vi "Formal Check Squares by Int.vi"(10 "Sudoku Formal In":T1, 11 "Sudoku Int":u8[][](array[numeric])) -> (2 "Sudoku Formal Out":T1, 3 "Is Modify":bool)   [LabVIEW 2015, in "Sudoku Library.lvlib"]
doc: "Created IvanLis by LabVIEW Portal\nProfile: http://labviewportal.org/memberlist.php?mode=viewprofile&u=987\neMail: IvanLisanov@gMail.com\nTelegram: https://t.me/IvanLis"
uses:
  Sudoku Library.lvlib
  TypeDef/Sudoku Formal.ctl
  TypeDef/Cell Formal.ctl
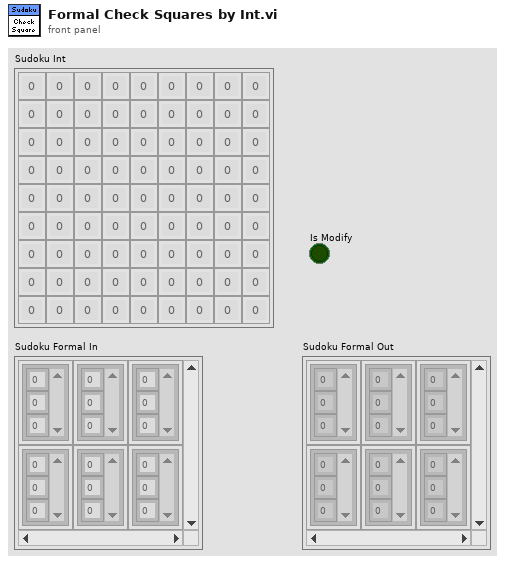
[diagram p1: front panel]
types:
  T1 = typedef "Sudoku Library.lvlib/Sudoku Formal.ctl" = T2[][]
  T2 = typedef "Sudoku Library.lvlib/Cell Formal.ctl" = cluster{"Variant":u8[]}
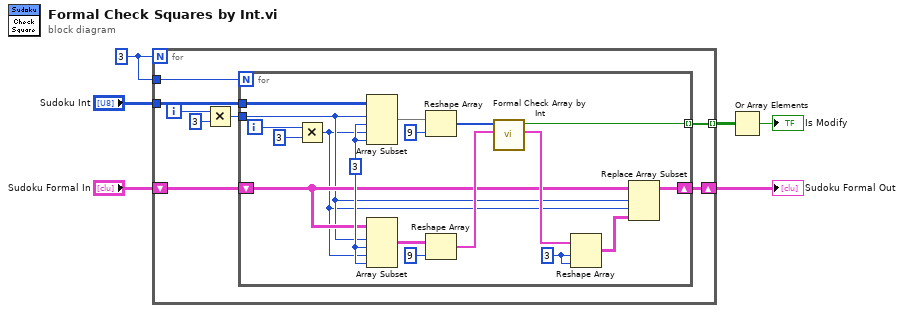
[diagram p0: block diagram]
diagram:
  w5 = 3
  n1 = for {
    N: w5 -> [_]
    tunnel: "Sudoku Int" -> [w14]
    tunnel: w5 -> [w13]
    tunnel: [w8] -> w3 mode=indexing
    shift-right: [w7] -> w1
    shift-left: "Sudoku Formal In" -> [w9]
    i -> [w12]
    n2 = Multiply(x=w12, y=3) -> (x*y=w10:i32)
    n3 = for {
      N: w13 -> [_]
      tunnel: w14 -> [w32]
      tunnel: w10 -> [w16]
      tunnel: [w22] -> w8 mode=indexing
      shift-right: [w18] -> w7
      shift-left: w9 -> [w19]
      i -> [w30]
      w20 = 3 ("dimension size")
      w27 = 3 ("y")
      n4 = Multiply(x=w30, y=3) -> (x*y=w15:i32)
      n5 = Array Subset(array=w32, index (row)=w16, length (row)=w27, index (col)=w15, length (col)=w27) -> (w29:u8[][])
      n6 = Array Subset(array=w19, index (row)=w16, length (row)=w27, index (col)=w15, length (col)=w27) -> (w25:T1)
      n7 = Reshape Array(w29, 9 ("dimension size")) -> (w24:u8[])
      n8 = Reshape Array(w25, 9 ("dimension size")) -> (w23:T2[])
      n9 = call "Formal Check Array by Int.vi"("Array Formal In"=w23, "Array In"=w24) -> ("Array Formal Out"=w21:T2[], "Is Modify"=w22:bool)  [unwired: 8 in]
      n10 = Reshape Array(w21, w20, w20) -> (w17:T2[][])
      n11 = Replace Array Subset(array=w19, new element=w17, index (row)=w16, index (col)=w15) -> (w18:T1)
    }
  }
  "Sudoku Formal Out" <- w1
  n12 = Or Array Elements(Boolean array=w3) -> (logical OR=→"Is Modify":bool)
